vi "Handle Request.vi"(7 "Processing In":refnum<class "Processing.lvclass">, 11 "HTTPS Redirect Handler in":refnum<class "HTTPS Redirect Handler.lvclass">) -> (0 "error out":errorcluster, 5 "Processing":refnum<class "Processing.lvclass">)   [LabVIEW 2020, in "HTTP Server.lvlib" / "HTTPS Redirect Handler.lvclass"]
uses:
  HTTPS Redirect Handler.lvclass
  Processing/Processing.lvclass
  Processing/Processing.lvclass/Processing.ctl
  lv-http-util/HTTP Utils/Redirect Response/Redirect Response.lvclass
  C:/dev/lv20CE/relink/lv-http-util/HTTP Utils/Response/Response.lvclass
  HTTPS Redirect Handler.lvclass/HTTPS Redirect Handler.ctl
  lv-http-util/HTTP Utils/Request/Request.lvclass
  Server/Server.lvclass
  lv-uri/URI/URI/URI.lvclass
  C:/dev/lv20CE/relink/lv-http-util/HTTP Utils/Redirect Response/Redirect Response.lvclass
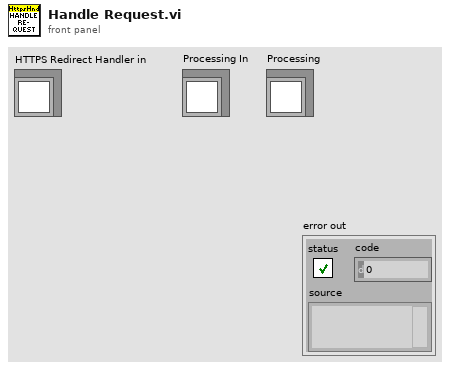
[diagram p1: front panel]
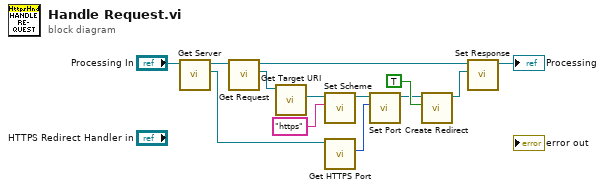
[diagram p0: block diagram]
diagram:
  n1 = call "Get Server.vi"("Processing in"="Processing In") -> ("Server"=w4:refnum<class "Server.lvclass">, "Processing out"=w5:refnum<class "Processing.lvclass">)  [unwired: 9 in]
  n2 = call "Get Request.vi"("Processing in"=w5) -> ("Request"=w13:refnum<class "Request.lvclass">, "Processing out"=w9:refnum<class "Processing.lvclass">)  [unwired: 9 in]
  n3 = call "Get Target URI.vi"("Request in"=w13) -> ("Target URI"=w12:refnum<class "URI.lvclass">)  [unwired: 8 in, 2 out]
  n4 = call "Set Scheme.vi"("Scheme"="https", "URI in"=w12) -> ("URI out"=w3:refnum<class "URI.lvclass">)  [unwired: 9 in]
  n5 = call "Get HTTPS Port.vi"("Server in"=w4) -> ("HTTPS Port"=w2:u16)  [unwired: 8 in, 2 out]
  n6 = call "Set Port.vi"("Port"=w2, "URI in"=w3) -> ("URI out"=w1:refnum<class "URI.lvclass">)  [unwired: 9 in]
  n7 = call "Create Redirect.vi"("Permanent? (F)"=TRUE, "Redirect URI"=w1) -> ("Redirect Response out"=w8:refnum<class "Redirect Response.lvclass">)  [unwired: 8 in, 1 out]
  n8 = call "Set Response.vi"("Response"=w8, "Processing in"=w9) -> ("Processing out"=→"Processing":refnum<class "Processing.lvclass">)  [unwired: 9 in]
